vi "ParameterChange_Wrapper.vi"(2 "Action":T1={"Macro Instructions"=[{"Duration (s)"=1.0, "Steps"=1, "Changes"=[TRUE, FALSE], "Triggers"=[FALSE, FALSE, FALSE, FALSE, FALSE, FALSE, FALSE, FALSE, FALSE, FALSE, FALSE, FALSE, TRUE, FALSE, FALSE, FALSE, FALSE, FALSE, FALSE, FALSE, FALSE, FALSE, FALSE, FALSE, FALSE, FALSE, FALSE, FALSE, FALSE, FALSE, FALSE, FALSE, FALSE, FALSE, FALSE, FALSE, FALSE, FALSE], "RAW cmds 2D"=[[0, 0, 0, 0, 0, 0, 0, 0], [0, 0, 0, 0, 0, 0, 0, 0]]}], "Slow AO Array"=[{"ao line"="ao0", "Duration, Gain, NewVal"=[0.0, 0.0]}, {"ao line"="ao1", "Duration, Gain, NewVal"=[0.0, 0.0]}, {"ao line"="ao2", "Duration, Gain, NewVal"=[0.0, 0.0]}, {"ao line"="0.000000E+0", "Duration, Gain, NewVal"=[0.0]}], "Duration (s)"=1.0, "Toggle"=FALSE} {"Slow AO Array"."Duration, Gain, NewVal" format="%#_3g"}, 3 "Tasks in":T4={"Outbits"="Outbits", "Counter"="Counter", "Digital Input Device"="6509", "Slow AO Device"="6723", "Fast AO"=["Fast AO_1", "Fast AO_2"], "Error Array"=[{"status"=FALSE, "code"=0, "source"=""}, {"status"=FALSE, "code"=0, "source"=""}, {"status"=FALSE, "code"=0, "source"=""}, {"status"=FALSE, "code"=0, "source"=""}], "outbits"=38, "inbits"=8}) -> (0 "inbit line":string, 1 "Wait for inbit":bool)   [LabVIEW 2018]
uses:
  Tasks_RT.ctl
  ActionCluster.ctl
  Instructions_RT.ctl
  ParameterSubCluster.ctl
panel:
  out "Duration (s)":dbl=1.0
  # "Tasks and errors"
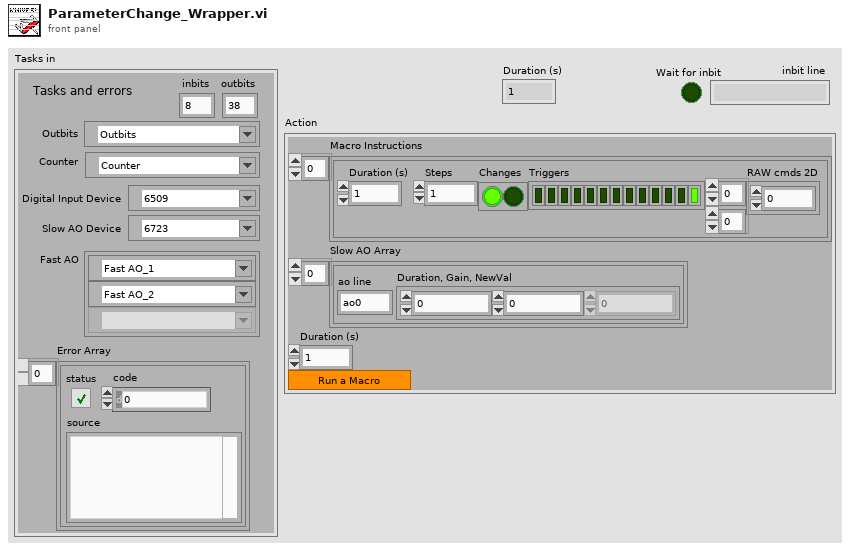
[diagram p1: front panel]
types:
  T1 = typedef "ActionCluster.ctl" = cluster{"Macro Instructions":T2, "Slow AO Array":T3, "Duration (s)":dbl, "Toggle":bool}
  T2 = typedef "Instructions_RT.ctl" = cluster{"Duration (s)":dbl, "Steps":i32, "Changes":bool[], "Triggers":bool[], "RAW cmds 2D":i16[][]}[]
  T3 = typedef "ParameterSubCluster.ctl" = cluster{"ao line":string, "Duration, Gain, NewVal":dbl[]}[]
  T4 = typedef "Tasks_RT.ctl" = cluster{"Outbits":refnum<k21>, "Counter":refnum<k21>, "Digital Input Device":tag, "Slow AO Device":tag, "Fast AO":refnum<k21>[], "Error Array":errorcluster[], "outbits":i32, "inbits":i32}
  T5 = cluster{"ao line":string, "Duration, Gain, NewVal":dbl[]}
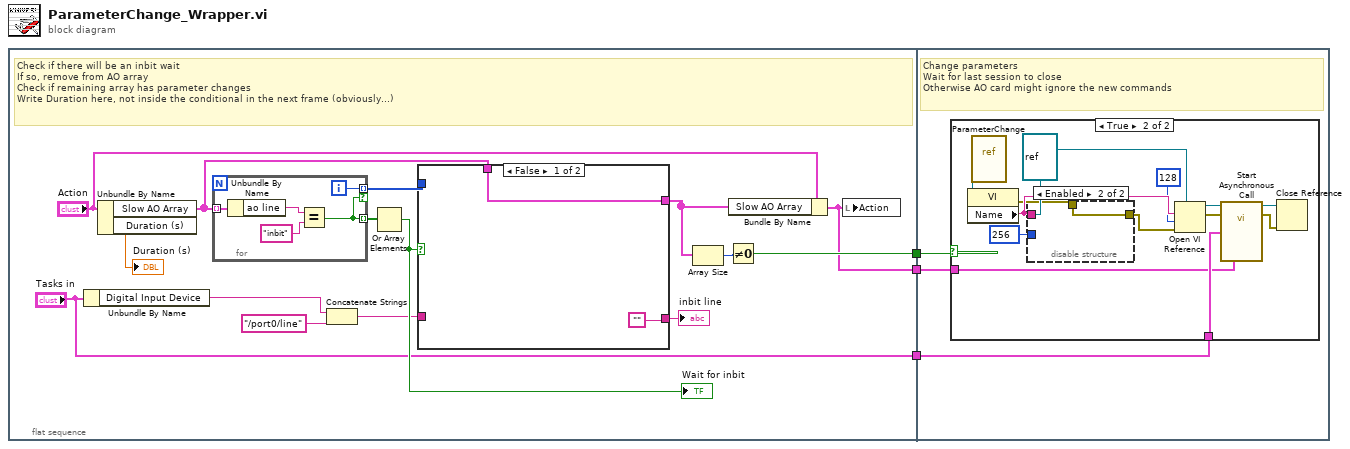
[diagram p0: block diagram]
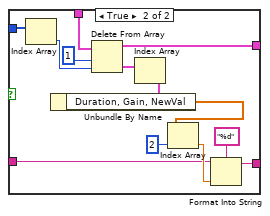
[diagram p2: hidden frame]
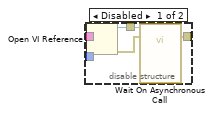
[diagram p4: hidden frame]
diagram:
  n1 = flat-sequence {
    tunnel: [w6] -> w3
    tunnel: [w5] -> w2
    tunnel: ["Tasks in"] -> w1
    tunnel: w3 -> [w41]
    tunnel: w2 -> [w40]
    tunnel: w1 -> [w39]
    frame #0 {
      # "Check if there will be an inbit wait\nIf so, remove from AO array\nCheck if remaining array has parameter changes\nWrite Duration here, not inside the conditional in the next frame (obviously...)"
      n2 = Unbundle By Name("Tasks in") -> ("Digital Input Device"=w8:tag)
      n3 = Unbundle By Name("Action") -> ("Slow AO Array"=w16:T3, "Duration (s)"=→"Duration (s)":dbl)
      n4 = for {
        tunnel: w16 -> [w38] mode=indexing
        tunnel: [w34] -> w18 mode=indexing
        tunnel: [w35] -> w17 mode=indexing if=w34
        i -> [w35]
        n5 = Unbundle By Name(w38) -> ("ao line"=w36:string)
        n6 = Equal?(x=w36, y="inbit") -> (x = y?=w34:bool)
      }
      n7 = Concatenate Strings(w8, "/port0/line" ("initial string")) -> (w9:string)
      n8 = Or Array Elements(Boolean array=w18) -> (logical OR=w12:bool)
      "Wait for inbit" <- w12
      n9 = case shown="False" w12 {
        tunnel: w17 -> [_ w33]
        tunnel: w16 -> [w20 w32]
        tunnel: [w20 w29] -> w14
        tunnel: ["" w22] -> w11
        tunnel: w9 -> [_ w23]
        frame False {
        }
        frame True {
          n10 = Index Array(array=w33) -> (element=w31:i32)  [unwired: 1 in]
          n11 = Delete From Array(array=w32, length=1, index=w31) -> (deleted portion=w28:T3, array with subset deleted=w29:T3)
          n12 = Index Array(array=w28) -> (element=w27:T5)  [unwired: 1 in]
          n13 = Unbundle By Name(w27) -> ("Duration, Gain, NewVal"=w26:dbl[])
          n14 = Index Array(array=w26, index=2) -> (element=w25:dbl)
          n15 = Format Into String(format string="%d", initial string=w23, w25) -> (resulting string=w22:string)  [unwired: 1 in, 1 out]
        }
      }
      "inbit line" <- w11
      n16 = Array Size(array=w14) -> (size(s)=w13:i32)
      n17 = Not Equal To 0?(x=w13) -> (x != 0?=w6:bool)
      n18 = Bundle By Name(cluster="Action", "Slow AO Array"=w14) -> (w5:T1)
      n19 = local write "Action"(w5) -> ()
    }
    frame #1 {
      # "Change parameters\nWait for last session to close\nOtherwise AO card might ignore the new commands"
      n20 = case shown="True" w41 {
        tunnel: w40 -> [_ w52]
        tunnel: w39 -> [_ w53]
        frame False {
        }
        frame True {
          w49 = refnum<vi> refnum ("type specifier VI Refnum (for type only)")
          n21 = vi-ref "ParameterChange.vi"() -> (w54:refnum<vi>)
          n22 = property class="VI"(reference=w54) -> (error out=w42:errorcluster, "Name"=w48:string)  [unwired: 1 in, 1 out]
          n23 = disable-structure shown="Enabled" {
            disable-tunnel: 256 ("options") -> [w60 _]
            disable-tunnel: [w59 w61] -> w50
            disable-tunnel: w49 -> [w57 _]
            disable-tunnel: w48 -> [w56 _]
            disable-tunnel: w42 -> [_ w61]
            frame Disabled {
              n24 = Open VI Reference(type specifier VI Refnum (for type only)=w57, vi path=w56, options=w60) -> (vi reference=w58:refnum<vi>, error out=w55:errorcluster)  [unwired: 3 in]
              n25 = call-by-ref "Wait On Asynchronous Call"(reference=w58, error in=w55) -> (error out=w59:errorcluster)  [unwired: 4 in, 1 out]
            }
            frame Enabled {
            }
          }
          n26 = Open VI Reference(type specifier VI Refnum (for type only)=w49, vi path=w48, options=128, error in (no error)=w50) -> (vi reference=w46:refnum<vi>, error out=w43:errorcluster)  [unwired: 2 in]
          n27 = call-by-ref "Start Asynchronous Call"(reference=w46, error in=w43, "Action"=w52, "Tasks in"=w53) -> (reference out=w44:refnum<vi>, error out=w45:errorcluster)  [unwired: 2 in]
          n28 = Close Reference(reference=w44, error in (no error)=w45) -> ()  [unwired: 1 out]
        }
      }
    }
  }
